vi "Wait for controller ready.vi"(0 "System no.":i32=1, 2 "Polling time, ms":i32=50, 5 "error in":errorcluster, 12 "Stop refnum":refnum<vi>) -> (15 "Stopped":bool, 19 "error out":errorcluster)   [LabVIEW 2020]
doc: "This VI waits for controller ready signal using #7 polling and stops also if Stop refnum or Local stop is TRUE, or if a communications error occured. Requires #7.vi to be present. When using as a sub-VI, use Stop refnum to stop VI from caller."
panel:
  in  "Local stop":bool
  # "This vi waits for controller ready signal using #7 \npolling and stops also if Stop refnum or Local stop\nis TRUE, or if a communications error occured."
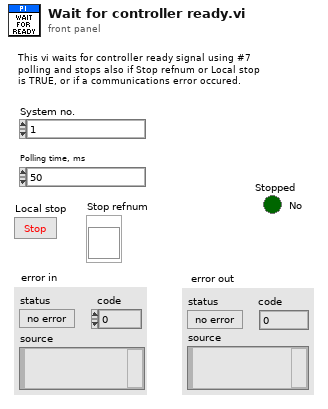
[diagram p1: front panel]
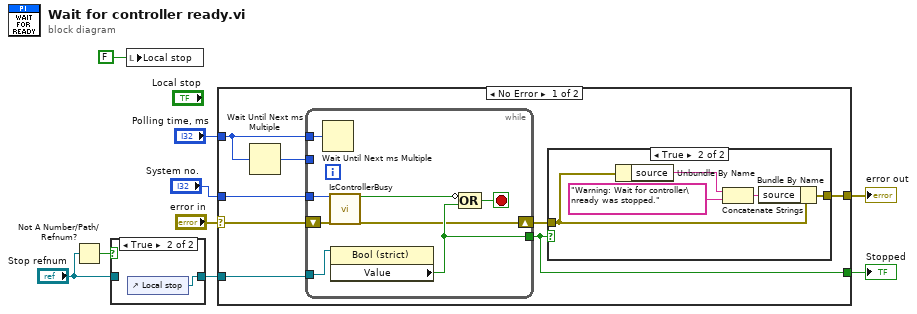
[diagram p0: block diagram]
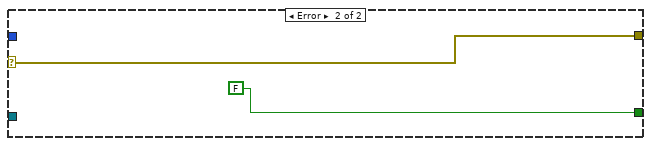
[diagram p4: hidden frame]
diagram:
  n1 = Not A Number/Path/Refnum?(number/path/refnum="Stop refnum") -> (NaN/Path/Refnum?=w6:bool)
  n2 = case shown="True" w6 {
    tunnel: [w10 w11] -> w4
    tunnel: "Stop refnum" -> [w10 _]
    frame False {
    }
    frame True {
      n3 = control-ref of="Local stop"() -> (w11:refnum<vi>)
    }
  }
  n4 = local write "Local stop"(FALSE ("Local stop")) -> ()
  n5 = case shown="No Error" "error in" {
    selector: "error in" -> [w12 w34]
    tunnel: [w16 w34] -> w9
    tunnel: w4 -> [w18 _]
    tunnel: [w15 FALSE] -> w7
    tunnel: "Polling time, ms" -> [w17 _]
    tunnel: "System no." -> [w13 _]
    frame No Error {
      n6 = Wait Until Next ms Multiple(millisecond multiple=w17) -> (millisecond timer value=w19:u32)
      n7 = while {
        tunnel: [w30] -> w15
        tunnel: w18 -> [w31]
        tunnel: w19 -> [_]
        tunnel: w13 -> [w33]
        shift-right: [w29] -> w14
        shift-left: w12 -> [w32]
        tunnel: w17 -> [w26]
        stop <- w27 stop-if-true
        n8 = Wait Until Next ms Multiple(millisecond multiple=w26) -> ()  [unwired: 1 out]
        n9 = call "IsControllerBusy.vi"("System no."=w33, "error in (no error)"=w32) -> ("Controller Busy"=w28:bool, "error out"=w29:errorcluster)  [unwired: 16 in]
        n10 = property class="Bool (strict)"(reference=w31) -> ("Value"=w30:bool)  [unwired: 1 in, 2 out]
        n11 = Compound Arithmetic op=OR(invert w28, w30) -> (w27:bool)
      }
      n12 = case shown="True" w15 {
        tunnel: [w20 w25] -> w16
        tunnel: w14 -> [w20 w23]
        frame False {
        }
        frame True {
          n13 = Unbundle By Name(w23) -> ("source"=w21:string)
          n14 = Concatenate Strings(w21, "Warning: Wait for controller\nready was stopped." ("source")) -> (w22:string)
          n15 = Bundle By Name(cluster=w23, "source"=w22) -> (w25:errorcluster)
        }
      }
    }
    frame Error {
    }
  }
  "error out" <- w9
  "Stopped" <- w7
